vi "Finish Round.vi"(6 "Turn Results In":T1, 7 "Round":u32, 9 "Teams In":refnum<class "Team.lvclass">[](array[class]), 11 "Map in":refnum<class "Map.lvclass">) -> (1 "Teams":refnum<class "Team.lvclass">[](array[class]), 3 "Map out":refnum<class "Map.lvclass">, 4 "Turn Results":T1)   [LabVIEW 2020, in "SquareBattle.lvlib" / "Map.lvclass"]
uses:
  Map.lvclass
  Turn Results.ctl
  Team/Team.lvclass
  Map.lvclass/Map.ctl
  SquareBattle.lvlib
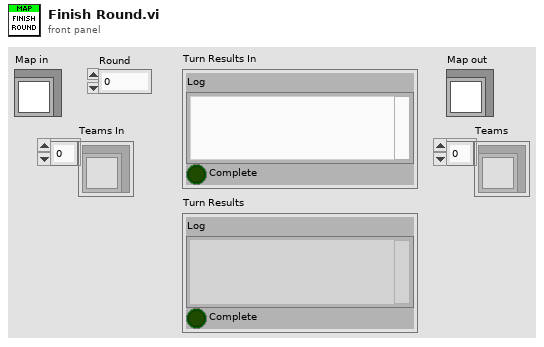
[diagram p1: front panel]
types:
  T1 = typedef "SquareBattle.lvlib/Turn Results.ctl" = cluster{"Log":string, "Complete":bool}
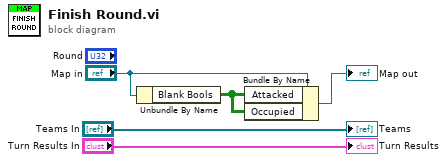
[diagram p0: block diagram]
diagram:
  n1 = Unbundle By Name("Map in") -> ("Blank Bools"=w3:bool[][])
  n2 = Bundle By Name(cluster="Map in", "Attacked"=w3, "Occupied"=w3) -> (→"Map out":refnum<class "Map.lvclass">)
  "Turn Results" <- "Turn Results In"
  "Teams" <- "Teams In"
